vi "FREQ_SPAN.vi"(7 "RO (T)":bool, 8 "error in":errorcluster {"code" format="%.0x"}, 10 "Span(MHz)":dbl, 11 "Session In":refnum<visa-resource-name>="GPIB0::16::INSTR") -> (0 "error out":errorcluster {"code" format="%.0x"}, 2 "Read Span (MHz)":dbl, 3 "Session Out":refnum<visa-resource-name>)   [LabVIEW 2018]
doc: "Launches the Instrument I/O Assistant, which you can use to communicate with message-based instruments and graphically parse the response. For example you can communicate with an instrument that uses a serial, Ethernet, or GPIB interface."
panel:
  in  "Timeout":u32=3000
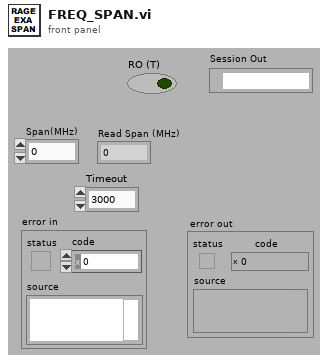
[diagram p1: front panel]
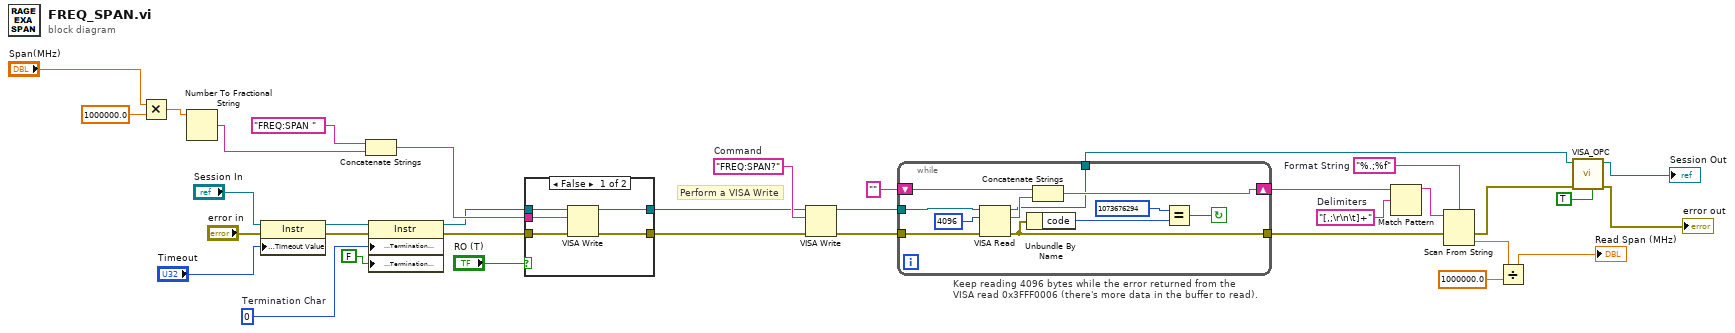
[diagram p0: block diagram]
diagram:
  w15 = "[,;\r\n\t]+"  # Delimiters
  w17 = "%.;%f"  # Format String
  w20 = "FREQ:SPAN?"  # Command
  w30 = u8 0  # Termination Char
  # "Keep reading 4096 bytes while the error returned from the\nVISA read 0x3FFF0006 (there's more data in the buffer to read)."
  # "Perform a VISA Write"
  n1 = Multiply(x="Span(MHz)", y=1000000.0) -> (x*y=w7:dbl)
  n2 = Number To Fractional String(number=w7) -> (F-format string=w6:string)  [unwired: 3 in]
  n3 = property class="Instr"(reference="Session In", error in="error in", "General Settings:Timeout Value"="Timeout") -> (reference out=w29:refnum<visa-resource-name>, error out=w32:errorcluster)
  n4 = Concatenate Strings("FREQ:SPAN " ("staticText"), w6) -> (w25:string)
  n5 = property class="Instr"(reference=w29, error in=w32, "Message Based Settings:Termination Character"=w30, "Message Based Settings:Termination Character Enable"=FALSE ("enable")) -> (reference out=w14:refnum<visa-resource-name>, error out=w31:errorcluster)
  n6 = case shown="False" "RO (T)" {
    tunnel: w31 -> [w40 w41]
    tunnel: [w39 w41] -> w26
    tunnel: w25 -> [w38 _]
    tunnel: w14 -> [w37 w42]
    tunnel: [w36 w42] -> w13
    frame False {
      n7 = VISA Write(VISA resource name=w37, write buffer=w38, error in (no error)=w40) -> (VISA resource name out=w36:refnum<visa-resource-name>, error out=w39:errorcluster)  [unwired: 1 out]
    }
    frame True {
    }
  }
  n8 = VISA Write(VISA resource name=w13, write buffer=w20, error in (no error)=w26) -> (VISA resource name out=w24:refnum<visa-resource-name>, error out=w23:errorcluster)  [unwired: 1 out]
  n9 = while {
    tunnel: w24 -> [w50]
    shift-right: [w44] -> w19
    shift-left: "" -> [w49]
    tunnel: w23 -> [w47]
    tunnel: [w46] -> w22
    tunnel: [w43] -> w4
    stop <- w45 continue-if-true
    n10 = VISA Read(VISA resource name=w50, byte count=u32 4096 ("byte count (0)"), error in (no error)=w47) -> (VISA resource name out=w43:refnum<visa-resource-name>, read buffer=w48:string, error out=w46:errorcluster)  [unwired: 1 out]
    n11 = Unbundle By Name(w46) -> ("code"=w52:i32)
    n12 = Concatenate Strings(w49, w48) -> (w44:string)
    n13 = Equal?(x=1073676294, y=w52) -> (x = y?=w45:bool)
  }
  n14 = Match Pattern(string=w19, regular expression=w15) -> (before substring=w18:string)  [unwired: 1 in, 3 out]
  n15 = Scan From String(format string=w17, input string=w18, error in=w22) -> (error out=w5:errorcluster, output 1=w16:dbl)  [unwired: 2 in, 2 out]
  n16 = Divide(x=w16, y=1000000.0) -> (x/y=→"Read Span (MHz)":dbl)
  n17 = call "VISA_OPC.vi"("OPC(T)"=TRUE ("OPC?(T)"), "error in"=w5, "Session In"=w4) -> ("error out"=→"error out":errorcluster, "Session Out"=→"Session Out":refnum<visa-resource-name>)  [unwired: 6 in, 1 out]
